vi "Save Sequence.vi"(8 "error in (no error)":errorcluster, 10 "#to save":u16=10, 11 "HIJ Vision Camera App in":refnum<class "HIJ Vision Camera App.lvclass">) -> (0 "error out":errorcluster, 3 "HIJ Vision Camera App out":refnum<class "HIJ Vision Camera App.lvclass">)   [LabVIEW 2020]
uses:
  HIJ Vision Camera App.lvclass/HIJ Vision Camera App.ctl
  HIJ Vision Camera App.lvclass
  C:/Users/AlexK/work/LabVIEW Programme/POLARIS CAM Log Abw und E/Submodules/HIJ Vision/Application Base Actors/HIJ Vision Application/HIJ Vision Application/HIJ Vision Application.lvclass
  C:/Users/AlexK/work/LabVIEW Programme/POLARIS CAM Log Abw und E/Submodules/Viewable Actor/ViewableActor/ViewableActor.lvclass
  C:/Program Files (x86)/National Instruments/LabVIEW 2020/vi.lib/ActorFramework/Actor/Actor.lvclass
  C:/Users/AlexK/work/LabVIEW Programme/POLARIS CAM Log Abw und E/Submodules/HIJ Vision/Analyze/Analyze Actor/IAnalysis/IAnalysis.lvclass
  C:/Users/AlexK/work/LabVIEW Programme/POLARIS CAM Log Abw und E/Submodules/HIJ Vision/Application Base Actors/HIJ Vision Camera App/HIJ Vision Camera App/HIJ Vision Camera App.lvclass
  C:/Users/AlexK/work/LabVIEW Programme/POLARIS CAM Log Abw und E/Submodules/HIJ Vision/Camera Actors/Camera Actor/ICamera/ICamera.lvclass
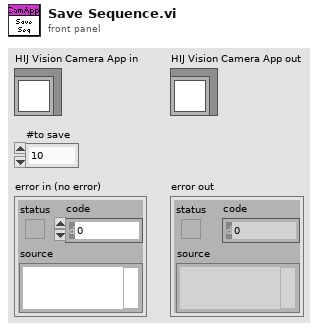
[diagram p1: front panel]
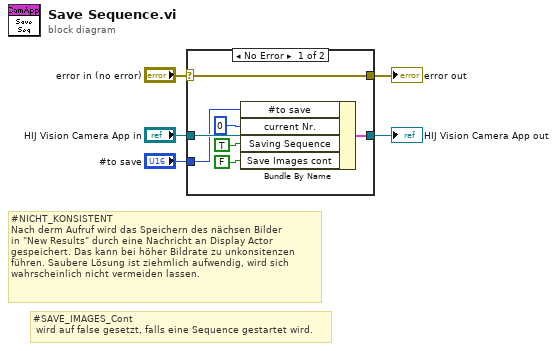
[diagram p0: block diagram]
diagram:
  # "#SAVE_IMAGES_Cont\n wird auf false gesetzt, falls eine Sequence gestartet wird."
  # "#NICHT_KONSISTENT\nNach derm Aufruf wird das Speichern des nächsen Bilder \nin \"New Results\" durch eine Nachricht an Display Actor \ngespeichert. Das kann bei höher Bildrate zu unkonsitenzen\nführen. Saubere Lösung ist ziehmlich aufwendig, wird sich \nwahrscheinlich nicht vermeiden lassen."
  n1 = case shown="No Error" "error in (no error)" {
    selector: "error in (no error)" -> [w11 w14]
    tunnel: [w11 w14] -> w4
    tunnel: [w10 w13] -> w2
    tunnel: "HIJ Vision Camera App in" -> [w12 w13]
    tunnel: "#to save" -> [w9 _]
    frame No Error {
      n2 = Bundle By Name(cluster=w12, "#to save"=w9, "current Nr."=0, "Saving Sequence"=TRUE, "Save Images cont"=FALSE) -> (w10:cluster{})
    }
    frame Error {
    }
  }
  "error out" <- w4
  "HIJ Vision Camera App out" <- w2
